vi "Get-Ball_Api.vi"(5 "障礙物位置2":enum16{"1-1", "1-2", "2-1", "2-2"}(ring), 6 "障礙物位置":enum16{"障礙物一", "障礙物二"}(ring), 7 "I2C Ref In":T2={"myRIO Reference"={"myRIO Model"=enum."Unknown", "myRIO Hardware Reference"={"Generic FPGA Reference"=refnum, "Allow multiple opens"=FALSE}}, "I2C Channels Enum"=enum."Not Connected", "I2C Configuration"={"I2C Transfer Rate"=enum."Fast mode (400 kbps)"}}, 8 "Error In":errorcluster, 9 "輸出顏色-位置":T1(array[cluster]), 10 "夾球開始位置":T10(ring), 11 "HiTechnicColorSensorV2 Ref":cluster{"I2C Ref Out":T2}) -> (0 "Error Out":errorcluster, 1 "輸出顏色-位置":T1(array[cluster]), 3 "HiTechnicColorSensorV2 Ref Out":cluster{"I2C Ref Out":T2})   [LabVIEW 2019]
uses:
  <vilib>/myRIO/Instrument Drivers/Onboard IO/I2C/typedefs/I2C Reference.ctl
  <vilib>/myRIO/Common/Instrument Driver Framework/Utilities/typedefs/myRIO Generic Hardware Reference.ctl
  <vilib>/myRIO/Common/Instrument Driver Framework/Utilities/typedefs/Hardware Version Enum.ctl
  <vilib>/myRIO/Common/Instrument Driver Framework/Utilities/typedefs/myRIO v1.0 Reference.ctl
  <vilib>/myRIO/Common/Instrument Driver Framework/Utilities/typedefs/Generic FPGA Reference.ctl
  <vilib>/myRIO/Common/Instrument Driver Framework/myRIO v1.0/I2C/typedefs/I2C Channels Enum.ctl
  <vilib>/myRIO/Instrument Drivers/Onboard IO/I2C/typedefs/I2C Configuration.ctl
  <vilib>/myRIO/Instrument Drivers/Onboard IO/I2C/typedefs/I2C Transfer Rate.ctl
  <vilib>/myRIO/Instrument Drivers/Onboard IO/I2C/I2C.lvlib
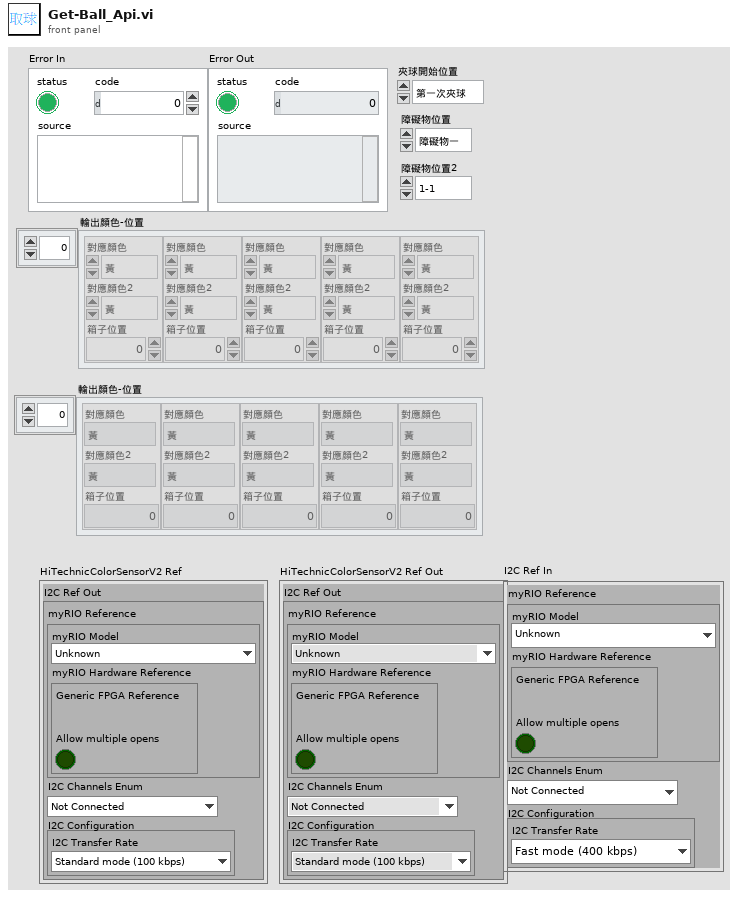
[diagram p1: front panel]
types:
  T1 = cluster{"對應顏色":enum16{"黃", "紅", "綠", "藍", "黑", "無"}, "對應顏色2":enum16{"黃", "紅", "綠", "藍", "黑", "無"}, "箱子位置":i32}[]
  T2 = typedef "I2C.lvlib/I2C Reference.ctl" = cluster{"myRIO Reference":T3, "I2C Channels Enum":T7, "I2C Configuration":T8}
  T3 = typedef "myRIO Generic Hardware Reference.ctl" = cluster{"myRIO Model":T4, "myRIO Hardware Reference":T5}
  T4 = typedef "Hardware Version Enum.ctl" = enum16{"Unknown", "myRIO-1900", "myRIO-1950", "roboRIO", "NI ELVIS RIO CM", "ELVIS III"}
  T5 = typedef "myRIO v1.0 Reference.ctl" = cluster{"Generic FPGA Reference":T6, "Allow multiple opens":bool}
  T6 = typedef "Generic FPGA Reference.ctl" = refnum<k20>
  T7 = typedef "I2C Channels Enum.ctl" = enum16{"Not Connected", "A/I2C", "B/I2C", "I2C/I2C"}
  T8 = typedef "I2C.lvlib/I2C Configuration.ctl" = cluster{"I2C Transfer Rate":T9}
  T9 = typedef "I2C.lvlib/I2C Transfer Rate.ctl" = enum16{"Standard mode (100 kbps)", "Fast mode (400 kbps)"}
  T10 = enum16{"第一次夾球", "第二次夾球", "第三次夾球", "第四次夾球", "第五次夾球"}
  T11 = enum16{"前", "後", "オ", "右", "無", "0", "1", "2", "3", "4", "5", "6", "7"}
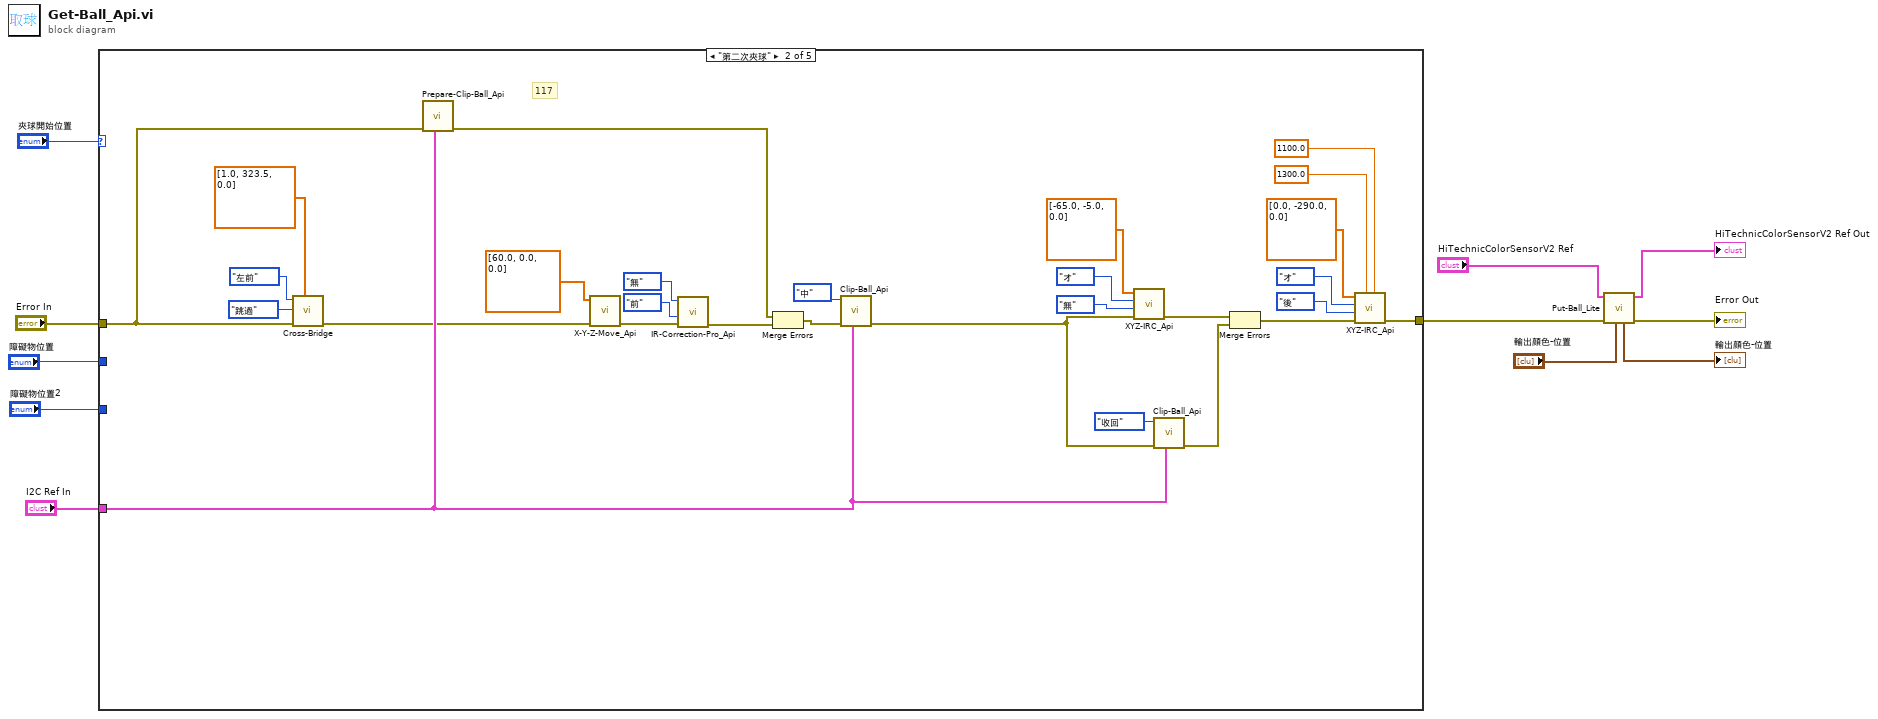
[diagram p0: block diagram]
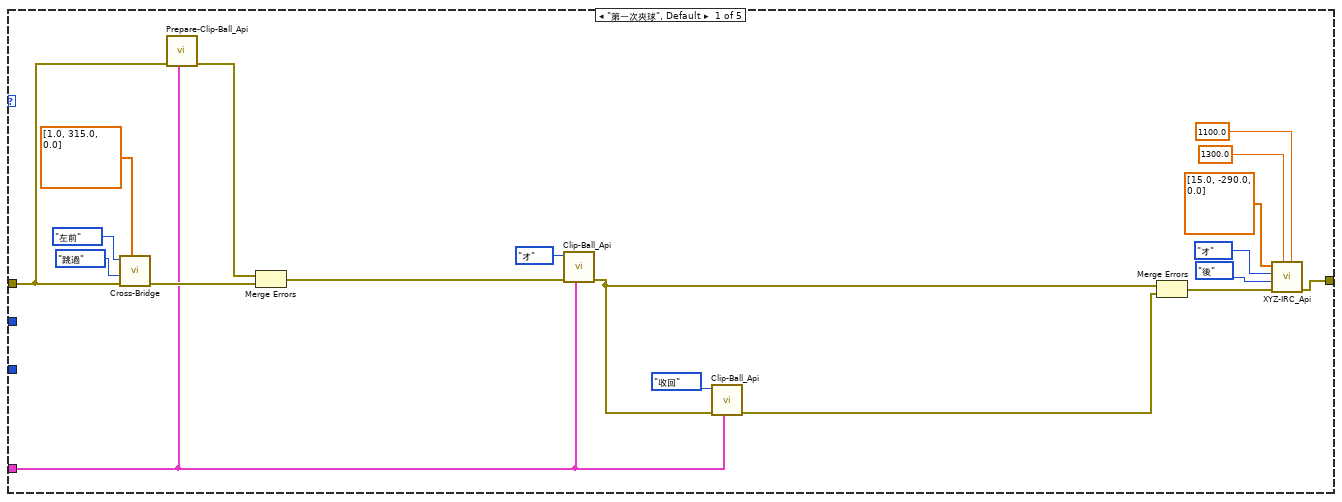
[diagram p2: hidden frame]
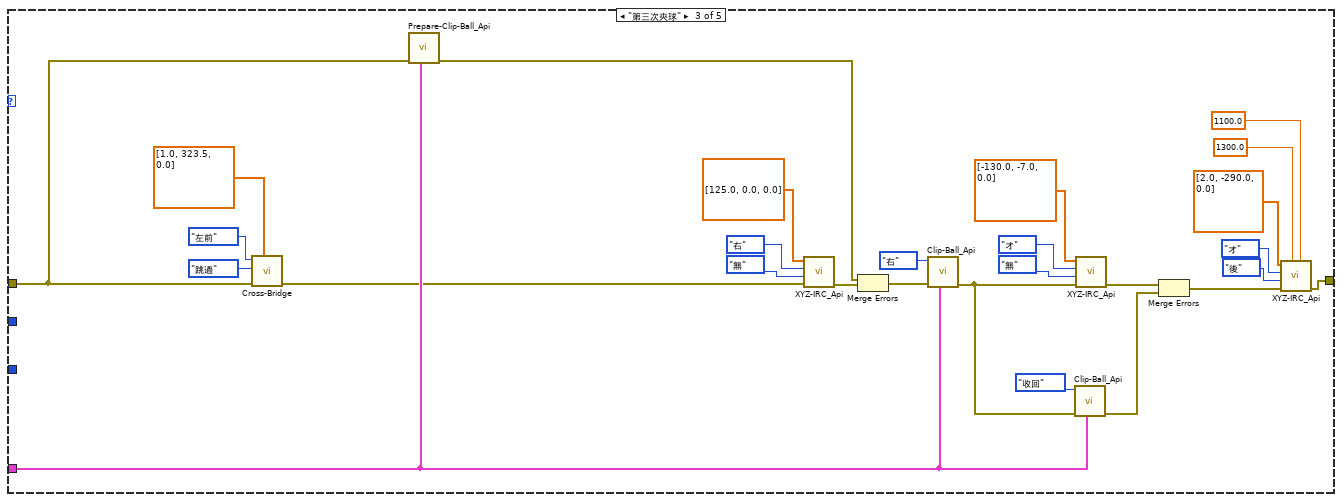
[diagram p3: hidden frame]
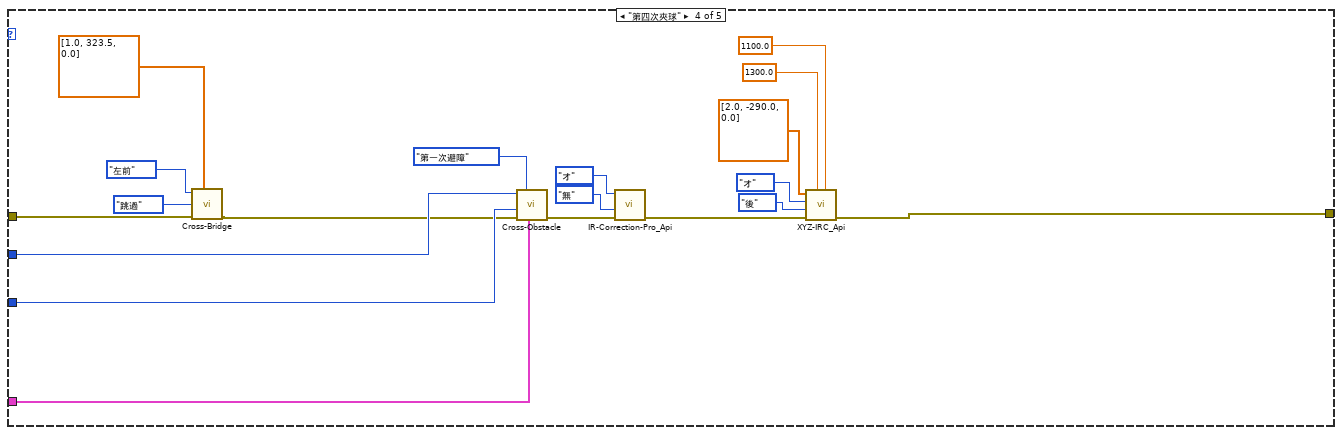
[diagram p4: hidden frame]
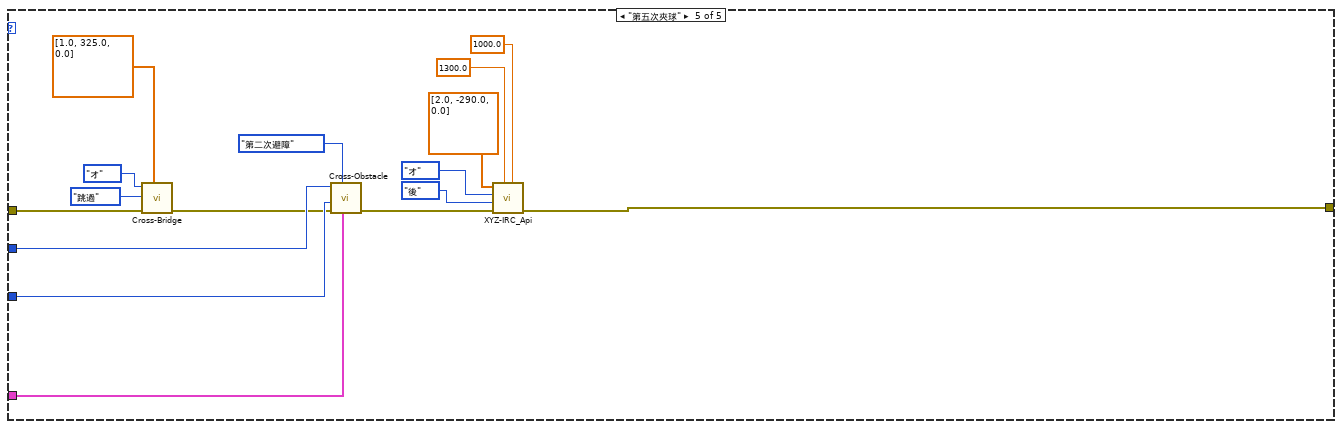
[diagram p5: hidden frame]
diagram:
  n1 = case shown="\"第二次夾球\"" "夾球開始位置" {
    tunnel: "Error In" -> [w22 w51 w69 w94 w110]
    tunnel: [w17 w48 w76 w93 w109] -> w6
    tunnel: "障礙物位置" -> [_ _ _ w104 w120]
    tunnel: "I2C Ref In" -> [w18 w49 w68 w103 w119]
    tunnel: "障礙物位置2" -> [_ _ _ w98 w115]
    frame "第一次夾球", Default {
      n2 = call "Cross-Bridge.vi"("X-Y-Z移動"=dbl[] [1.0, 315.0, 0.0], "Error In"=w22, "動作"=enum16{"補後退", "跳過"}."跳過", "校正選擇"=enum16{"左前", "オ"}."左前") -> ("Error Out"=w21:errorcluster)  [unwired: 7 in]
      n3 = call "Prepare-Clip-Ball_Api.vi"("I2C Ref In"=w18, "Error In"=w22) -> ("Error Out"=w23:errorcluster)  [unwired: 9 in]
      n4 = Merge Errors(w23, w21) -> (w13:errorcluster)
      n5 = call "Clip-Ball_Api.vi"("I2C Ref In"=w18, "Error In"=w13, "動作"=enum16{"オ", "中", "右", "收回", "合併"}."オ") -> ("Error Out"=w12:errorcluster)  [unwired: 8 in]
      n6 = call "Clip-Ball_Api.vi"("I2C Ref In"=w18, "Error In"=w12, "動作"=enum16{"オ", "中", "右", "收回", "合併"}."收回") -> ("Error Out"=w16:errorcluster)  [unwired: 8 in]
      n7 = Merge Errors(w12, w16) -> (w15:errorcluster)
      n8 = call "XYZ-IRC_Api.vi"("加速度"=1100.0, "最高速"=1300.0, "Error"=w15, "副邊校正"=T11."後", "主編校正"=enum16{"前", "後", "オ", "右", "無"}."オ", "X-Y-Z移動"=dbl[] [15.0, -290.0, 0.0]) -> ("Error Out"=w17:errorcluster)  [unwired: 5 in]
    }
    frame "第二次夾球" {
      # "117"
      n9 = call "Cross-Bridge.vi"("X-Y-Z移動"=dbl[] [1.0, 323.5, 0.0], "Error In"=w51, "動作"=enum16{"補後退", "跳過"}."跳過", "校正選擇"=enum16{"左前", "オ"}."左前") -> ("Error Out"=w39:errorcluster)  [unwired: 7 in]
      n10 = call "Prepare-Clip-Ball_Api.vi"("I2C Ref In"=w49, "Error In"=w51) -> ("Error Out"=w34:errorcluster)  [unwired: 9 in]
      n11 = call "X-Y-Z-Move_Api.vi"("Error In"=w39, "X-Y-Z移動"=dbl[] [60.0, 0.0, 0.0]) -> ("Error Out"=w41:errorcluster)  [unwired: 8 in, 1 out]
      n12 = call "IR-Correction-Pro_Api.vi"("Error In"=w41, "副邊校正"=T11."前", "主編校正"=enum16{"前", "後", "オ", "右", "無"}."無") -> ("Error Out"=w33:errorcluster)  [unwired: 8 in]
      n13 = Merge Errors(w34, w33) -> (w35:errorcluster)
      n14 = call "Clip-Ball_Api.vi"("I2C Ref In"=w49, "Error In"=w35, "動作"=enum16{"オ", "中", "右", "收回", "合併"}."中") -> ("Error Out"=w32:errorcluster)  [unwired: 8 in]
      n15 = call "XYZ-IRC_Api.vi"("Error"=w32, "副邊校正"=T11."無", "主編校正"=enum16{"前", "後", "オ", "右", "無"}."オ", "X-Y-Z移動"=dbl[] [-65.0, -5.0, 0.0]) -> ("Error Out"=w47:errorcluster)  [unwired: 7 in]
      n16 = call "Clip-Ball_Api.vi"("I2C Ref In"=w49, "Error In"=w32, "動作"=enum16{"オ", "中", "右", "收回", "合併"}."收回") -> ("Error Out"=w46:errorcluster)  [unwired: 8 in]
      n17 = Merge Errors(w47, w46) -> (w45:errorcluster)
      n18 = call "XYZ-IRC_Api.vi"("加速度"=1100.0, "最高速"=1300.0, "Error"=w45, "副邊校正"=T11."後", "主編校正"=enum16{"前", "後", "オ", "右", "無"}."オ", "X-Y-Z移動"=dbl[] [0.0, -290.0, 0.0]) -> ("Error Out"=w48:errorcluster)  [unwired: 5 in]
    }
    frame "第三次夾球" {
      n19 = call "Cross-Bridge.vi"("X-Y-Z移動"=dbl[] [1.0, 323.5, 0.0], "Error In"=w69, "動作"=enum16{"補後退", "跳過"}."跳過", "校正選擇"=enum16{"左前", "オ"}."左前") -> ("Error Out"=w59:errorcluster)  [unwired: 7 in]
      n20 = call "Prepare-Clip-Ball_Api.vi"("I2C Ref In"=w68, "Error In"=w69) -> ("Error Out"=w66:errorcluster)  [unwired: 9 in]
      n21 = call "XYZ-IRC_Api.vi"("Error"=w59, "副邊校正"=T11."無", "主編校正"=enum16{"前", "後", "オ", "右", "無"}."右", "X-Y-Z移動"=dbl[] [125.0, 0.0, 0.0]) -> ("Error Out"=w62:errorcluster)  [unwired: 7 in]
      n22 = Merge Errors(w66, w62) -> (w67:errorcluster)
      n23 = call "Clip-Ball_Api.vi"("I2C Ref In"=w68, "Error In"=w67, "動作"=enum16{"オ", "中", "右", "收回", "合併"}."右") -> ("Error Out"=w82:errorcluster)  [unwired: 8 in]
      n24 = call "Clip-Ball_Api.vi"("I2C Ref In"=w68, "Error In"=w82, "動作"=enum16{"オ", "中", "右", "收回", "合併"}."收回") -> ("Error Out"=w73:errorcluster)  [unwired: 8 in]
      n25 = call "XYZ-IRC_Api.vi"("Error"=w82, "副邊校正"=T11."無", "主編校正"=enum16{"前", "後", "オ", "右", "無"}."オ", "X-Y-Z移動"=dbl[] [-130.0, -7.0, 0.0]) -> ("Error Out"=w61:errorcluster)  [unwired: 7 in]
      n26 = Merge Errors(w61, w73) -> (w72:errorcluster)
      n27 = call "XYZ-IRC_Api.vi"("加速度"=1100.0, "最高速"=1300.0, "Error"=w72, "副邊校正"=T11."後", "主編校正"=enum16{"前", "後", "オ", "右", "無"}."オ", "X-Y-Z移動"=dbl[] [2.0, -290.0, 0.0]) -> ("Error Out"=w76:errorcluster)  [unwired: 5 in]
    }
    frame "第四次夾球" {
      n28 = call "Cross-Bridge.vi"("X-Y-Z移動"=dbl[] [1.0, 323.5, 0.0], "Error In"=w94, "動作"=enum16{"補後退", "跳過"}."跳過", "校正選擇"=enum16{"左前", "オ"}."左前") -> ("Error Out"=w86:errorcluster)  [unwired: 7 in]
      n29 = call "Cross-Obstacle.vi"("I2C Ref In"=w103, "避障回數"=enum16{"第一次避障", "第二次避障"}."第一次避障", "Error In"=w86, "障礙物位置2"=w98, "障礙物位置"=w104) -> ("Error Out"=w101:errorcluster)  [unwired: 6 in]
      n30 = call "IR-Correction-Pro_Api.vi"("Error In"=w101, "副邊校正"=T11."無", "主編校正"=enum16{"前", "後", "オ", "右", "無"}."オ") -> ("Error Out"=w92:errorcluster)  [unwired: 8 in]
      n31 = call "XYZ-IRC_Api.vi"("加速度"=1100.0, "最高速"=1300.0, "Error"=w92, "副邊校正"=T11."後", "主編校正"=enum16{"前", "後", "オ", "右", "無"}."オ", "X-Y-Z移動"=dbl[] [2.0, -290.0, 0.0]) -> ("Error Out"=w93:errorcluster)  [unwired: 5 in]
    }
    frame "第五次夾球" {
      n32 = call "Cross-Bridge.vi"("X-Y-Z移動"=dbl[] [1.0, 325.0, 0.0], "Error In"=w110, "動作"=enum16{"補後退", "跳過"}."跳過", "校正選擇"=enum16{"左前", "オ"}."オ") -> ("Error Out"=w108:errorcluster)  [unwired: 7 in]
      n33 = call "Cross-Obstacle.vi"("I2C Ref In"=w119, "避障回數"=enum16{"第一次避障", "第二次避障"}."第二次避障", "Error In"=w108, "障礙物位置2"=w115, "障礙物位置"=w120) -> ("Error Out"=w113:errorcluster)  [unwired: 6 in]
      n34 = call "XYZ-IRC_Api.vi"("加速度"=1000.0, "最高速"=1300.0, "Error"=w113, "副邊校正"=T11."後", "主編校正"=enum16{"前", "後", "オ", "右", "無"}."オ", "X-Y-Z移動"=dbl[] [2.0, -290.0, 0.0]) -> ("Error Out"=w109:errorcluster)  [unwired: 5 in]
    }
  }
  n35 = call "Put-Ball_Lite.vi"("輸出顏色-位置"="輸出顏色-位置", "Error In"=w6, "HiTechnicColorSensorV2 Ref In"="HiTechnicColorSensorV2 Ref") -> ("Error Out"=→"Error Out":errorcluster, "HiTechnicColorSensorV2 Ref Out"=→"HiTechnicColorSensorV2 Ref Out":cluster{"I2C Ref Out":T2}, "輸出顏色-位置"=→"輸出顏色-位置":T1)  [unwired: 6 in]
